vi "to string array.vi"(8 "error in (no error)":errorcluster, 11 "module configuration in":refnum<class "SystemLink configuration.lvclass">) -> (0 "error out":errorcluster, 1 "Array":string[][](array[string]), 2 "version":string, 3 "module configuration out":refnum<class "SystemLink configuration.lvclass">)   [LabVIEW 2015, in "SystemLink configuration.lvclass"]
uses:
  SystemLink configuration.lvclass
  SystemLink configuration.lvclass/SystemLink configuration.ctl
  <vilib>/NI/Tag Bus/tag/tag descriptor.lvclass/tag descriptor.ctl
  <vilib>/NI/Tag Bus Module Framework/channel/TBM channel.lvclass/TBM channel.ctl
  Read Lines.vi
  <vilib>/NI/Tag Bus Module Framework/channel/TBM channel.lvclass
  <vilib>/NI/Tag Bus/tag/tag descriptor.lvclass
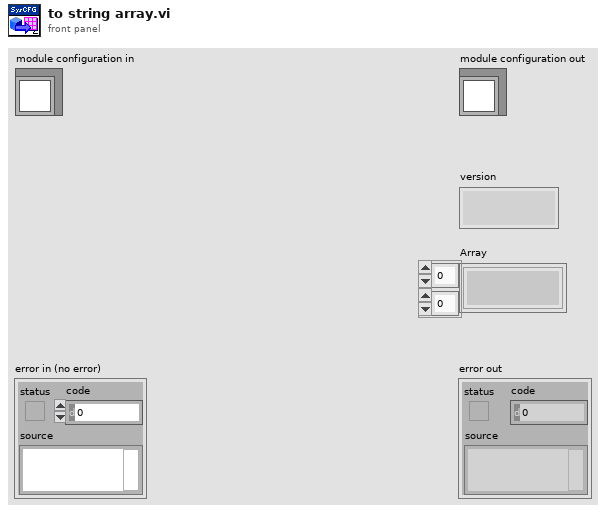
[diagram p1: front panel]
types:
  T1 = typedef "SystemLink configuration.lvclass/Line.ctl" = cluster{"channel":refnum<class "TBM channel.lvclass">, "Data Tag Type":T2}
  T2 = typedef "SystemLink configuration.lvclass/Data Tag Type.ctl" = enum16{"Double", "Single", "I32", "I16", "I8", "U64", "U32", "U16", "U8", "Boolean", "String", "Timestamp"}
  T3 = typedef "TBM channel.lvclass/channel classification.ctl" = enum16{"input data", "output data", "processing parameter", "processing result"}
  T4 = typedef "SystemLink configuration.lvclass/permissions.ctl" = enum32{"Read from SystemLink", "Write to SystemLink"}
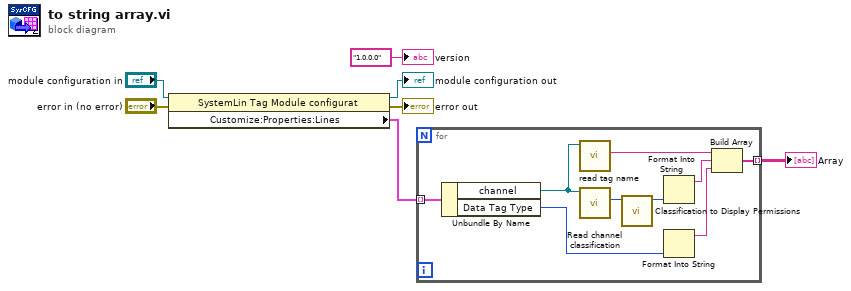
[diagram p0: block diagram]
diagram:
  n1 = property class="SystemLin Tag Module configurat"(reference="module configuration in", error in="error in (no error)") -> (reference out=→"module configuration out":refnum<class "SystemLink configuration.lvclass">, error out=→"error out":errorcluster, "Customize:Properties:Lines"=w4:T1[])
  n2 = for {
    tunnel: w4 -> [w16] mode=indexing
    tunnel: [w9] -> w3 mode=indexing
    n3 = Unbundle By Name(w16) -> ("channel"=w11:refnum<class "TBM channel.lvclass">, "Data Tag Type"=w8:T2)
    n4 = call <vilib>:"read tag name.vi"("system tag in"=w11) -> ("name"=w15:string)  [unwired: 8 in, 2 out]
    n5 = call <vilib>:"Read channel classification.vi"("channel in"=w11) -> ("channel classification"=w14:T3)  [unwired: 8 in, 2 out]
    n6 = call "Classification to Display Permissions.vi"("channel classification"=w14) -> ("permissions"=w13:T4)  [unwired: 10 in]
    n7 = Format Into String(w13) -> (resulting string=w12:string)  [unwired: 3 in, 1 out]
    n8 = Format Into String(w8) -> (resulting string=w10:string)  [unwired: 3 in, 1 out]
    n9 = Build Array(w15, w12, w10) -> (w9:string[])
  }
  "Array" <- w3
  "version" <- "1.0.0.0" ("version")
